vi "Read-all-gui-parameters.vi"(8 "error in":errorcluster, 11 "Filter params. ref. in":refnum<data-value>) -> (0 "error IO":errorcluster, 2 "Filter params.":T1, 3 "Filter params. ref.":refnum<data-value>)   [LabVIEW 2013, in "CameraVision.lvlib" / "CV-Filter.lvclass"]
uses:
  CV-Filter.lvclass
  Filter-parameters-gui.ctl
  Filter-settings.ctl
  Filter-characteristic.ctl
  Filter-apply.ctl
  CV-Filter.lvclass/CV-Filter.ctl
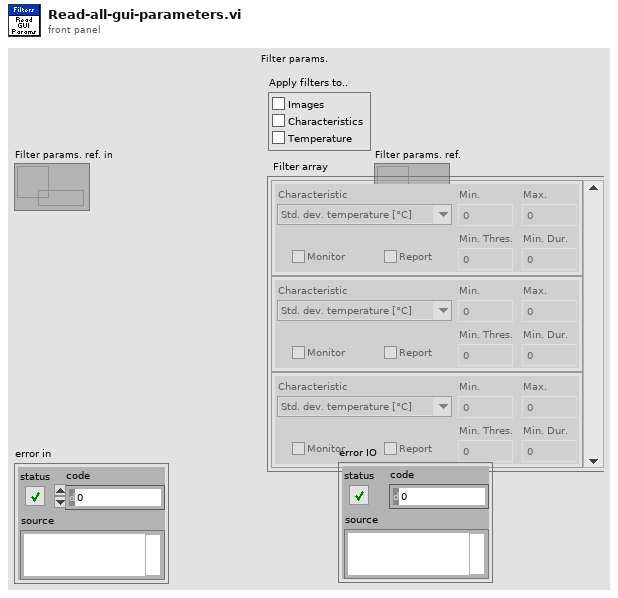
[diagram p1: front panel]
types:
  T1 = typedef "CameraVision.lvlib/CV-Filter.lvclass/Filter-parameters-gui.ctl" = cluster{"Filter array":T2[], "Storage filters":T4}
  T2 = typedef "CameraVision.lvlib/CV-Filter.lvclass/Filter-settings.ctl" = cluster{"Characteristic":T3, "Monitor":bool, "Min.":dbl, "Max.":dbl, "Min. Thres.":dbl, "Min. Dur.":u16, "Report":bool}
  T3 = typedef "CameraVision.lvlib/CV-Filter.lvclass/Filter-characteristic.ctl" = enum16{"Average intensity [0-255]", "Peak intensity [0-255]", "Melt-pool size [mm²]", "Melt-pool aspect ratio []", "Melt-pool fragments []", "Melt-pool position X [pixel]", "Melt-pool position Y [pixel]", "Average temperature [°C]", "Max. temperature [°C]", "Min. temperature [°C]", "Std. dev. temperature [°C]"}
  T4 = typedef "CameraVision.lvlib/CV-Filter.lvclass/Filter-apply.ctl" = cluster{"Filter images":bool, "Filter characteristics":bool, "Filter temperature":bool}
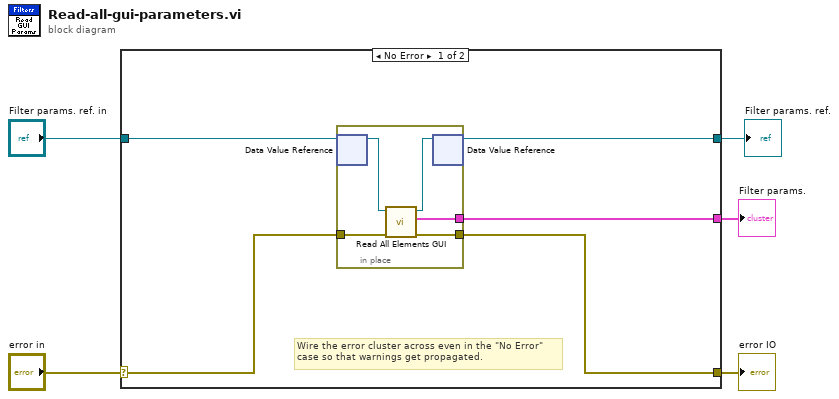
[diagram p0: block diagram]
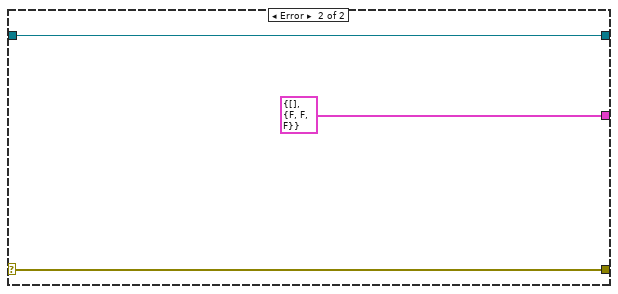
[diagram p2: hidden frame]
diagram:
  n1 = case shown="No Error" "error in" {
    selector: "error in" -> [w10 w18]
    tunnel: [w8 w18] -> w1
    tunnel: "Filter params. ref. in" -> [w7 w17]
    tunnel: [w9 T1 {"Filter array"=[], "Storage filters"={"Filter images"=FALSE, "Filter characteristics"=FALSE, "Filter temperature"=FALSE}} ("Alert params.")] -> w3
    tunnel: [w6 w17] -> w4
    frame No Error {
      # "Wire the error cluster across even in the \"No Error\"\ncase so that warnings get propagated."
      n2 = in-place {
        in-place-border: w10 -> [w15]
        in-place-border: [w13] -> w9
        in-place-border: [w14] -> w8
        n3 = in-place-dvr #1(w7) -> (w11:refnum<class "CV-Filter.lvclass">)  [unwired: 1 out]
        n4 = call "Read All Elements GUI.vi"("error in (no error)"=w15, "Filter params in"=w11) -> ("error out"=w14:errorcluster, "Filter params."=w13:T1, "Filter params out"=w12:refnum<class "CV-Filter.lvclass">)  [unwired: 7 in]
        n5 = in-place-dvr #1(w12) -> (w6:refnum<data-value>)  [unwired: 1 out]
      }
    }
    frame Error {
    }
  }
  "Filter params. ref." <- w4
  "Filter params." <- w3
  "error IO" <- w1
